vi "Read Waveforms.vi"   [LabVIEW 2023, in "Keysight-DSQx3014T.lvlib"]
doc: "Reads waveforms data."
uses:
  Keysight-DSQx3014T.lvlib
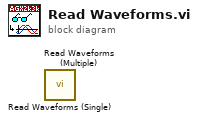
[diagram p0: block diagram]
diagram:
  n1 = call "Read Waveforms (Single).vi"() -> ()  [unwired: 9 in, 3 out]
  n2 = call "Read Waveforms (Multiple).vi"() -> ()  [unwired: 9 in, 3 out]
